vi "Actor Core.vi"(8 "error in":errorcluster, 11 "Nested in":refnum<class "Chat Window Controller UI.lvclass">) -> (0 "error out":errorcluster, 3 "Actor out":refnum<class "Actor.lvclass">)   [LabVIEW 2020, in "Chat Window UI.lvlib" / "Chat Window Controller UI.lvclass"]
doc: "(<B>Filename</B>: Actor Framework.lvlib:Actor.lvclass:Actor Core.vi)\n\nReceives messages to the actor, reacts to them, and initiates any error handling that may shut the actor down.\n\nDescendant classes may override this VI to append parallel tasks for the actor to complete while it handles messages. Overrides use the Call Parent Method node."
uses:
  Chat Window Controller UI.lvclass
  F:/Gitlab Repository/LabVIEW-Study/10.Top 5 Actor Framework Overrides/Chat Room with Interface/Chat Window UI Controller/Chat Window UI Controller/Chat Window UI Controller.lvclass
  C:/Program Files (x86)/National Instruments/LabVIEW 2020/vi.lib/ActorFramework/Actor/Actor.lvclass
  <vilib>/ActorFramework/Actor/Actor.lvclass
  Chat Window Controller UI.lvclass/Chat Window Controller UI.ctl
  Chat Window UI Controller/Chat Window UI Controller/Chat Window UI Controller.lvclass/Chat Window UI Controller.ctl
  <vilib>/ActorFramework/Actor/Actor.lvclass/Actor.ctl
  <vilib>/ActorFramework/Message Enqueuer/Message Enqueuer.lvclass/Message Enqueuer.ctl
  Application Control/Message.ctl
  Chat Window UI Controller/Chat Window UI Controller Messages/Send message Msg/Send message Msg.lvclass/Send message Msg.ctl
  Chat Window UI Controller/Chat Window UI Controller Messages/Own Status Change Msg/Own Status Change Msg.lvclass/Own Status Change Msg.ctl
  <vilib>/ActorFramework/Message Enqueuer/Init from Existing Queue.vi
  <vilib>/ActorFramework/Message Enqueuer/Enqueue.vi
  <vilib>/ActorFramework/Stop Msg/Stop Msg.lvclass
  C:/Program Files (x86)/National Instruments/LabVIEW 2020/vi.lib/ActorFramework/Message/Message.lvclass
  Chat Window UI Controller/Chat Window UI Controller Messages/Send message Msg/Send message Msg.lvclass
  Chat Window UI Controller/Chat Window UI Controller Messages/Own Status Change Msg/Own Status Change Msg.lvclass
  <vilib>/ActorFramework/Message Priority Queue/Priority Enqueue.vi
  Chat Window UI Controller/Chat Window UI Controller/Chat Window UI Controller.lvclass
  <vilib>/ActorFramework/Message Enqueuer/Message Enqueuer.lvclass
  F:/Gitlab Repository/LabVIEW-Study/10.Top 5 Actor Framework Overrides/Chat Room with Interface/Chat Window UI/Chat Window Controller UI.lvclass
panel:
  out "Online Status List":string[](array[string])
  in  "Send Message":bool
  in  "Direct Message":string
  in  "To":string(combo)
  out "Messages Log":string
  in  "My Status":string
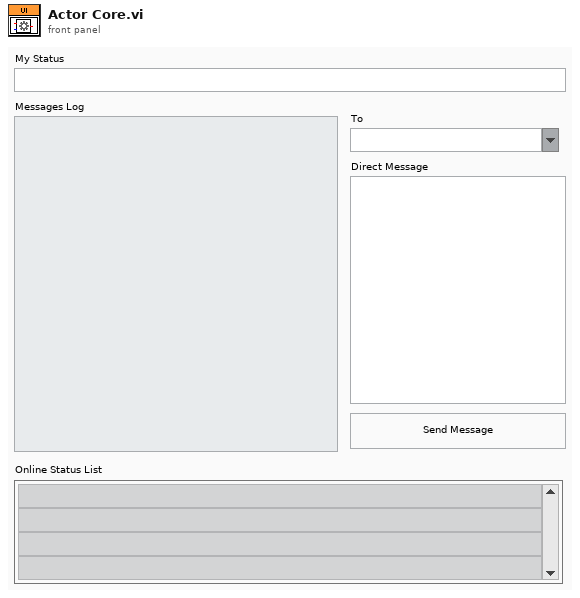
[diagram p1: front panel]
types:
  T1 = cluster{"Stop":refnum<user-event>, "On Line Status":refnum<user-event>, "Messages Log":refnum<user-event>}
  T2 = typedef "Message.ctl" = cluster{"From":string, "To":string, "Message":string}
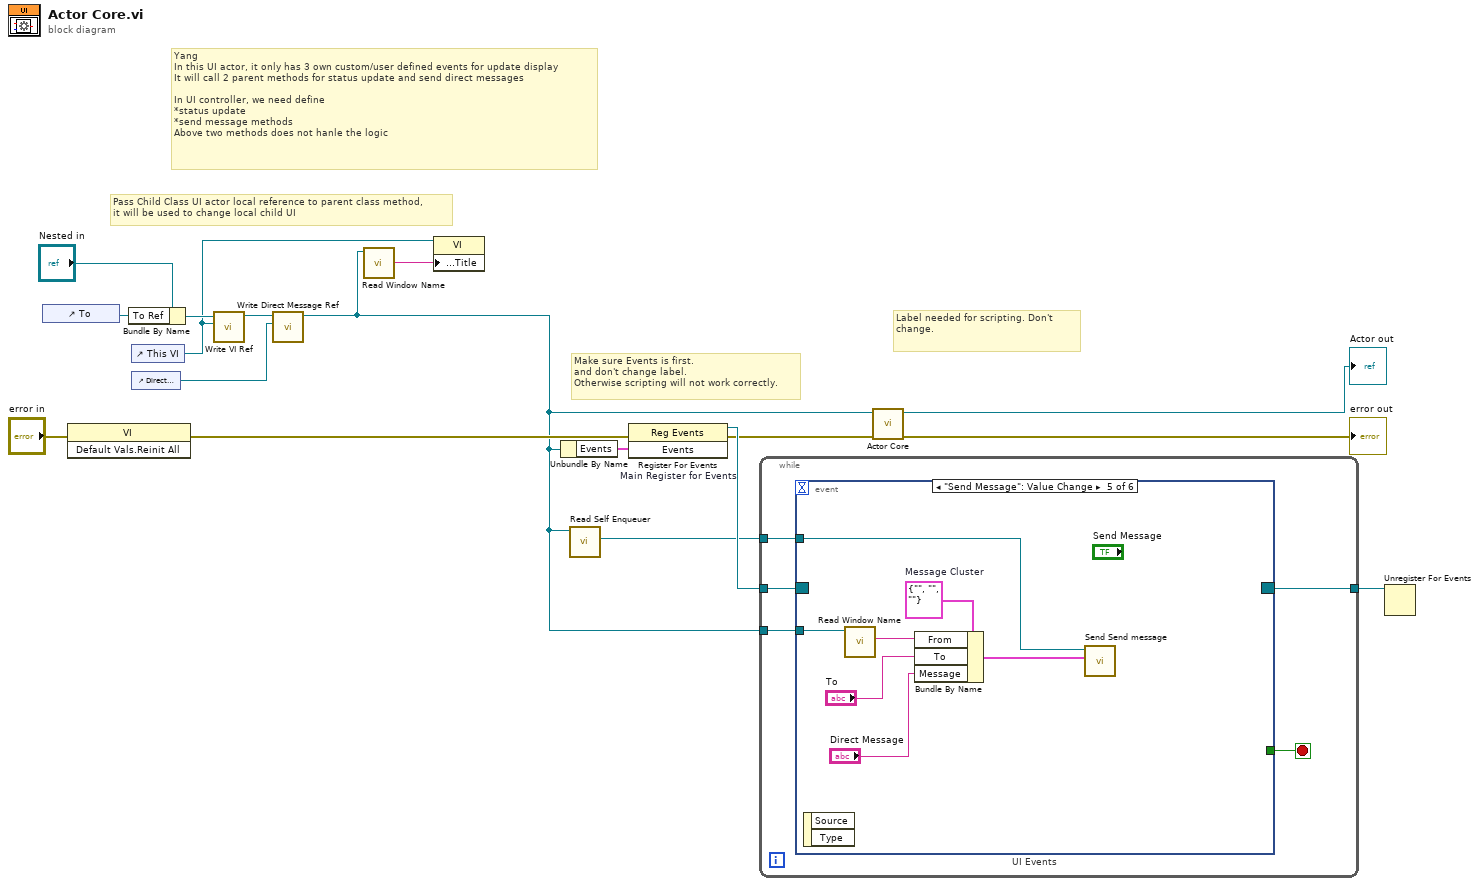
[diagram p0: block diagram]
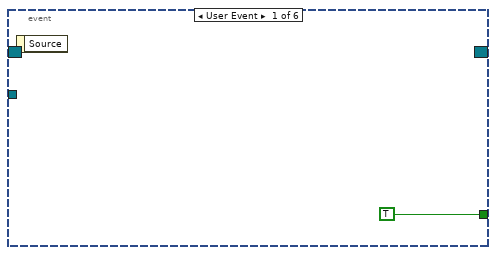
[diagram p2: hidden frame]
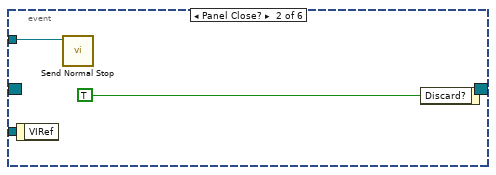
[diagram p3: hidden frame]
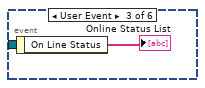
[diagram p4: hidden frame]
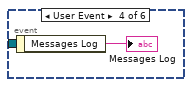
[diagram p5: hidden frame]
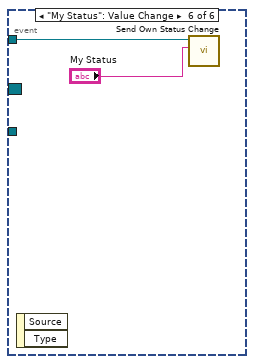
[diagram p6: hidden frame]
diagram:
  # "Pass Child Class UI actor local reference to parent class method, \nit will be used to change local child UI"
  # "Yang\nIn this UI actor, it only has 3 own custom/user defined events for update display \nIt will call 2 parent methods for status update and send direct messages \n\nIn UI controller, we need define \n*status update\n*send message methods  \nAbove two methods does not hanle the logic"
  # "Label needed for scripting. Don't change."
  # "Make sure Events is first.\nand don't change label.\nOtherwise scripting will not work correctly."
  n1 = control-ref of="To"() -> (w7:refnum<vi>)
  n2 = invoke class="VI" method="Default Vals.Reinit All"(error in="error in") -> (error out=w9:errorcluster)  [unwired: 2 in, 2 out]
  n3 = Bundle By Name(cluster="Nested in", "To Ref"=w7) -> (w6:refnum<class "Chat Window Controller UI.lvclass">)
  n4 = control-ref of="This VI"() -> (w3:refnum<vi>)
  n5 = control-ref of="Direct Message"() -> (w1:refnum<vi>)
  n6 = call "Write VI Ref.vi"("VI Ref"=w3, "Chat Window Controller in"=w6) -> ("Chat Window Controller out"=w5:refnum<class "Chat Window Controller UI.lvclass">)  [unwired: 8 in, 1 out]
  n7 = call "Write Direct Message Ref.vi"("Direct Message"=w1, "Chat Window Controller in"=w5) -> ("Chat Window Controller out"=w2:refnum<class "Chat Window Controller UI.lvclass">)  [unwired: 8 in, 1 out]
  n8 = call "Read Window Name.vi"("Chat Window Controller in"=w2) -> ("Window Name"=w4:string)  [unwired: 8 in, 2 out]
  n9 = property class="VI"(reference=w3, "Front Panel.Title"=w4) -> ()  [unwired: 1 in, 2 out]
  n10 = Unbundle By Name(w2) -> ("Events"=w14:T1)
  n11 = call <vilib>:"Read Self Enqueuer.vi"("Actor"=w2) -> ("Self Enqueuer"=w12:refnum<class "Message Enqueuer.lvclass">)  [unwired: 10 in]
  n12 = register-events "Main Register for Events"(error in=w9, w14) -> (reference out=w15:refnum<event-registration>, error out=w11:errorcluster)  [unwired: 1 in]
  n13 = while {
    tunnel: w15 -> [w22]
    tunnel: [w20] -> w13
    tunnel: w12 -> [w19]
    tunnel: w2 -> [w18]
    stop <- w21 stop-if-true
    n14 = event "UI Events" shown="[4] \"Send Message\": Value Change" {
      selector: w22 -> [_ _ _ _ _ _]
      dyn-events: [_ _ _ _ _ _] -> w20
      timeout: _ -> [_ _ _ _ _ _]
      tunnel: [TRUE _ _ _ _ _] -> w21
      tunnel: w19 -> [_ w24 _ _ w30 w36]
      tunnel: w18 -> [_ _ _ _ w28 _]
      event User Event {
        n15 = event-data() -> ()  [unwired: 1 in, 1 out]
      }
      event Panel Close? {
        n16 = event-data() -> ()  [unwired: 1 in, 1 out]
        n17 = call <vilib>:"Send Normal Stop.vi"("Message Enqueuer"=w24) -> ()  [unwired: 10 in, 1 out]
        n18 = event-data("Discard?"=TRUE) -> ()  [unwired: 1 in, 1 out]
      }
      event User Event {
        n19 = event-data() -> ("On Line Status"=→"Online Status List":string[])  [unwired: 1 in]
      }
      event User Event {
        n20 = event-data() -> ("Messages Log"=→"Messages Log":string)  [unwired: 1 in]
      }
      event "Send Message": Value Change {
        w34 = T2 {"From"="", "To"="", "Message"=""}  # Message Cluster
        n21 = event-data() -> ()  [unwired: 1 in, 2 out]
        n22 = call "Read Window Name.vi"("Chat Window Controller in"=w28) -> ("Window Name"=w33:string)  [unwired: 8 in, 2 out]
        n23 = Bundle By Name(cluster=w34, "From"=w33, "To"="To", "Message"="Direct Message") -> (w29:T2)
        n24 = call "Send Send message.vi"("Message Queue"=w29, "Message Enqueuer"=w30) -> ()  [unwired: 8 in, 2 out]
      }
      event "My Status": Value Change {
        n25 = event-data() -> ()  [unwired: 1 in, 2 out]
        n26 = call "Send Own Status Change.vi"("New Status"="My Status", "Message Enqueuer"=w36) -> ()  [unwired: 8 in, 2 out]
      }
    }
  }
  n27 = call-parent "Actor Core.vi"("error in"=w11, "Chat Window Controller in"=w2) -> ("error out"=→"error out":errorcluster, "Actor out"=→"Actor out":refnum<class "Actor.lvclass">)  [unwired: 8 in]
  n28 = Unregister For Events(event registration refnum=w13) -> ()  [unwired: 1 in, 1 out]
